vi "ReadByID.vi"(0 "reference in":refnum<class "UDS.lvclass">, 1 "ID":u16=13680 format="%.0x", 5 "error in (no error)":errorcluster) -> (14 "reference out":refnum<class "UDS.lvclass">, 15 "DID":u8[](array[numeric]) format="%.0x", 19 "error out":errorcluster)   [LabVIEW 2020, in "UDS.lvclass"]
uses:
  UDS.lvclass
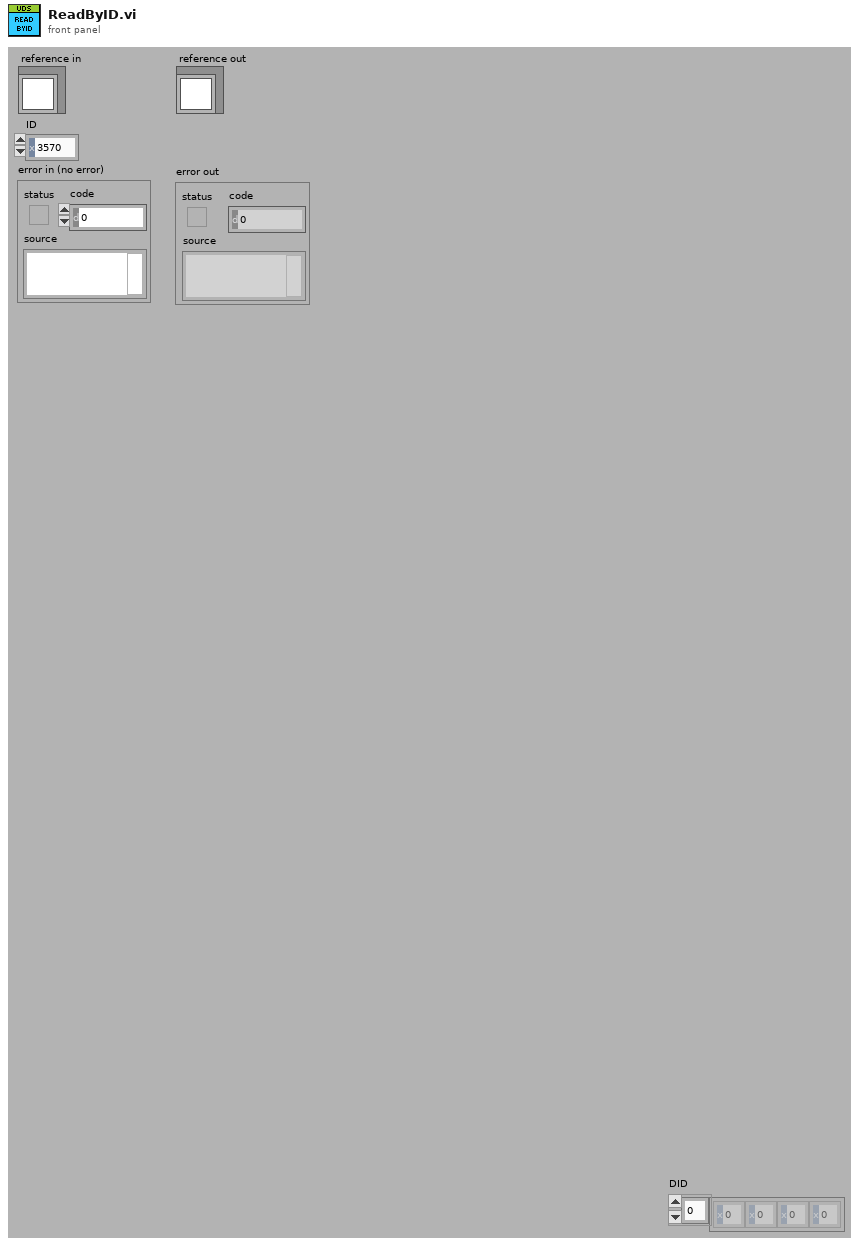
[diagram p1: front panel]
types:
  T1 = typedef "UDS.lvclass/ObjectAttributesRef.ctl" = refnum<data-value>
  T2 = typedef "UDS.lvclass/ObjectAttributes.ctl" = cluster{"MyAttribute":dbl, "UDSSetting":cluster{"InterfacName":string, "Baud Rate":u64, "FD Baud Rate":u64, "Transport Protocol":T3, "IO Mode":u32, "Max DLC":u16, "Transmit ID":u32, "Receive ID":u32, "Wait Time CF (STmin)":u32, "Fill Byte":u32}, "diag ref":T4}
  T3 = typedef "NI_Automotive Diagnostic Command Set.lvlib/Transport Protocol Selector.ctl" = enum16{"ISO TP - Normal Mode", "ISO TP - Mixed Mode", "VW TP 2.0", "Diagnostics on IP", "ISO TP LIN"}
  T4 = typedef "NI_Automotive Diagnostic Command Set.lvlib/Diag Reference.ctl" = cluster{"Diag CAN Handle":u32, "Transport Protocol":T3, "Receive Address Extension":u8, "Transmit Address Extension":u8, "Receive CAN Id":u32, "Transmit CAN Id":u32, "Log Frames ?":bool, "My TP Address":u8, "Other TP Address":u8, "T1":u16, "T2":u16, "T3":u16, "T4":u16, "Tx SN":u8, "Block Size":u8, "Rx SN":u8, "VW TP Initialized?":bool, "Tx block no":u8, "baud rate":u64, "Interface":string, "Channel Diag CAN Handle":u32, "UDP Connection ID":refnum<k16>, "TCP Connection ID":refnum<k5>, "Target IP Addr":u32, "Source Address":u16, "Target Address":u16, "Send Header NACK?":bool, "DLL Handle":u32, "NAD":u8, "Time Stamp read first":dbl, "Time Stamp read last":dbl, "Time Stamp write first":dbl, "Time Stamp write last":dbl, "Time Stamp write":dbl, "Time Stamp read":dbl, " I/O Mode":u32, "FD Baudrate":u64, "TX_DL":u16, "RX_DL":u16, "DoIP Protocol Version":T5, " Selected I/O Mode":u32, "TesterPresent Counter":u32, "TesterPresent Limit":u32, "TesterPresent Tick[ms]":i32, "TesterPresent RequireResponse?":bool, "TesterPresent Stored Ref?":bool, "TesterPresent Message":u8[], "TesterPresent Task Handle":i32, "TesterPresent Semaphore":T6, "Response Plausibility Check":u32, "Default Version?":bool, "Diagostic Globals":T7, "Session-based Properties?":bool}
  T5 = typedef "NI_Automotive Diagnostic Command Set.lvlib/DoIP Protocol Version.ctl" = u8
  T6 = typedef "Semaphore RefNum" = refnum<k1>
  T7 = typedef "NI_Automotive Diagnostic Command Set.lvlib/Diag Globals.ctl" = cluster{"Timeout FC (Bs)":u32, "Timeout CF (Cr)":u32, "Timeout Diag Command":u32, "Receive Block Size (BS)":u8, "Wait Time CF (STmin)":u8, "Max Waits (N_WFTmax)":u8, "Waits to Send (N_WAIT)":i32, "Time between Waits (TW)":u32, "Fill CAN Frames?":bool, "Fill Byte":u32, "Invalid Response as Error?":bool, "Max RspPending Count":u32, "VWTP Command Timeout":u32, "Transport Protocol":T3, "Diag CAN Handle":u32, "DLL Handle":u32, "Timeout RspPending":u32}
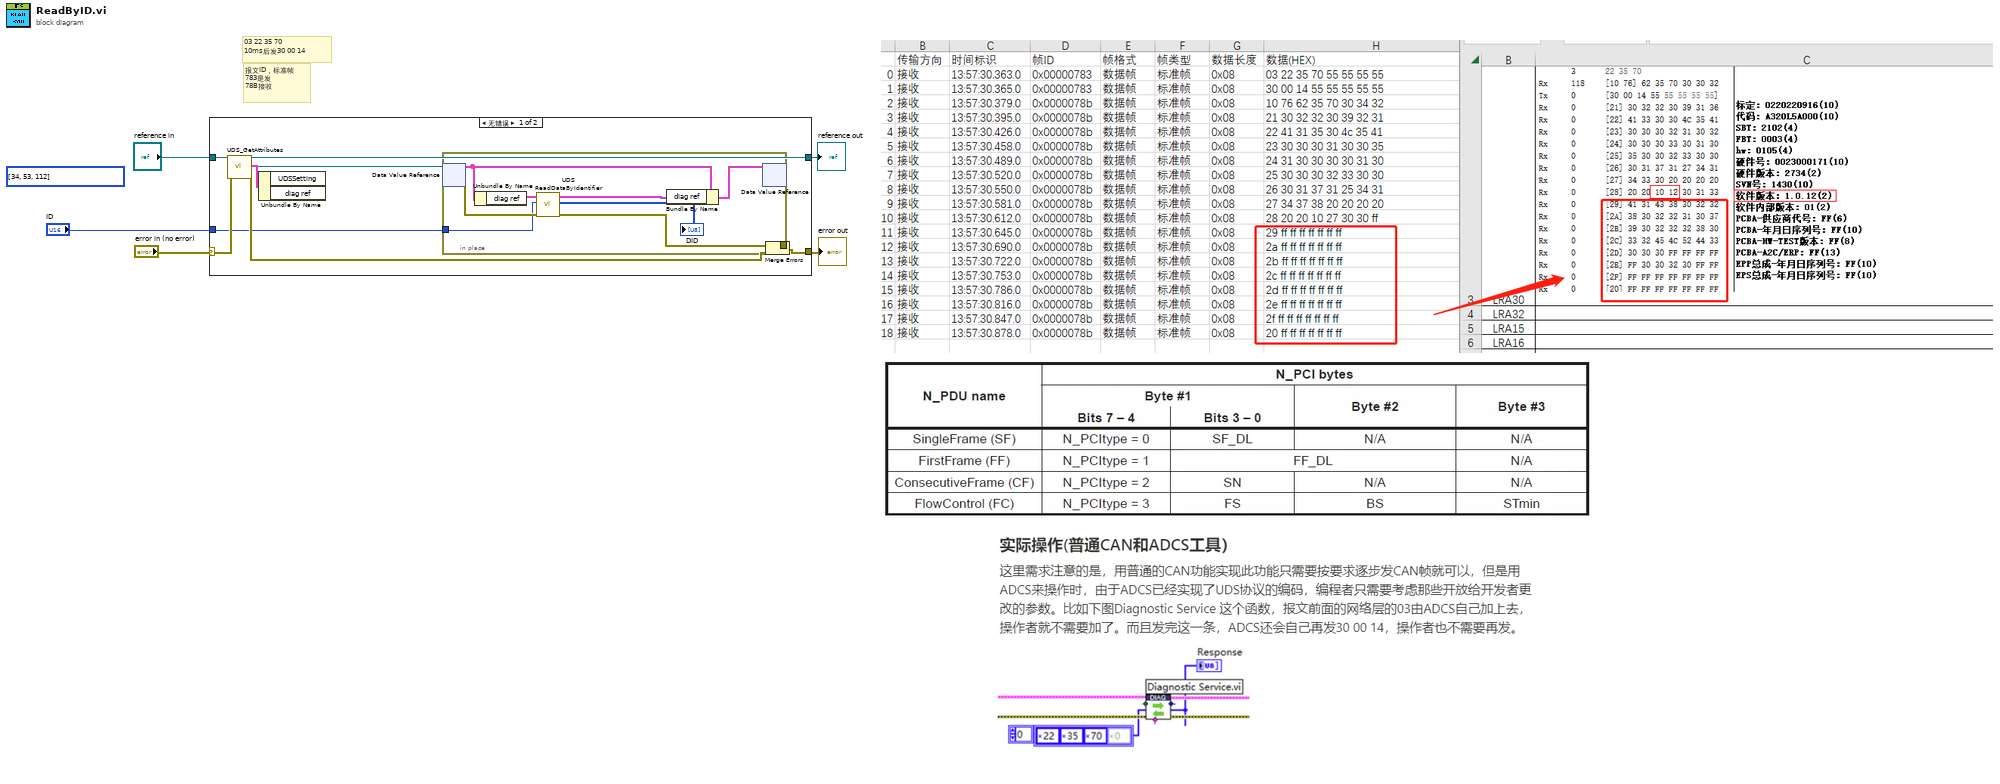
[diagram p0: block diagram]
diagram:
  (unwired) u8[] [34, 53, 112] ("Request")
  # "03 22 35 70     \n10ms后发30 00 14"
  # "报文ID，标准帧\n783是发\n78B接收"
  n1 = case shown="无错误" "error in (no error)" {
    selector: "error in (no error)" -> [w14 w24]
    tunnel: [w10 w24] -> w4
    tunnel: [w13 w23] -> w2
    tunnel: "reference in" -> [w11 w23]
    tunnel: "ID" -> [w6 _]
    frame No Error {
      n2 = call "UDS_GetAttributes.vi"("reference in"=w11, "error in (no error)"=w14) -> ("reference out"=w13:refnum<class "UDS.lvclass">, "attributes ref"=w9:T1, "attributes"=w12:T2, "error out"=w7:errorcluster)  [unwired: 14 in]
      n3 = Unbundle By Name(w12) -> ()  [unwired: 2 out]
      n4 = in-place {
        in-place-border: [w17] -> w8
        in-place-border: w6 -> [w16]
        n5 = in-place-dvr #1(w9) -> (w21:T2, w18:errorcluster)
        n6 = Unbundle By Name(w21) -> ("diag ref"=w22:T4)
        n7 = call <vilib>:"UDS ReadDataByIdentifier.vi"("error in (no error)"=w18, "ID"=w16, "diag ref in"=w22) -> ("error out"=w17:errorcluster, "data out"=→"DID":u8[], "diag ref out"=w20:T4)  [unwired: 5 in, 1 out]
        n8 = Bundle By Name(cluster=w21, "diag ref"=w20) -> (w19:T2)
        n9 = in-place-dvr #1(w19) -> ()  [unwired: 2 out]
      }
      n10 = Merge Errors(w8, w7) -> (w10:errorcluster)
    }
    frame Error {
    }
  }
  "error out" <- w4
  "reference out" <- w2
